vi "Day 4-2.vi"() -> ()   [LabVIEW 2019, in "Day 4.lvlib"]
uses:
  Day 4.lvlib
panel:
  out "Result":i32
  out "Winner Turn Number":i32
  out "Winner Board Status":bool[][](array[boolean])
  out "Winner Board":i32[][](array[numeric])
  in  "String":string="62,55,98,93,48,28,82,78,19,96,31,42,76,25,34,4,18,80,66,6,14,17,57,54,90,27,40,47,9,36,97,56,87,61,91,1,64,71,99,38,70,5,94,85,49,59,69,26,21,60,0,79,2,95,11,84,20,24,8,51,46,44,88,22,16,53,7,32,89,67,15,86,41,92,10,77,68,63,43,75,33,30,81,37,83,3,39,65,12,45,23,73,72,29,52,58,35,50,13,74\n\n10 83 98 12 33\n38 68  2 99 85\n16 89 54 50 97\n31  8 17 11 76\n 0 55 66 32 87\n\n77 60 61 59 16\n17 46 97  9 73\n42 82 25 32 29\n48 94 52 55 50\n95 14 67 79 34\n\n 6 31  5 74 67\n76 89 15 78 47\n54 49 62 32 38\n35 43 61 22 58\n75 97 33  8 16\n\n37 58 22 47 30\n 4 86 77 42 54\n73 94 87 34 55\n72 53 14 64 88\n23 21 36 52 66\n\n59 16 18 85 93\n96 56 50 53 94\n68 95 77  0 27\n47 30 88 46 65\n75 82 41 31 23\n\n88 96 94 75  3\n31 26 74 90 36\n59 22 41 84 54\n 6 68 37 20 93\n10 66 46  9 79\n\n33 78 12 62 73\n18 37  7 44 66\n69 15 54 53 82\n98 20 30 58 81\n56 95 36 91 99\n\n47 89 86 58 43\n49 72 84 94 51\n69 73 15 50  0\n46 81 76 31 61\n96 91 56  2 34\n\n22 91 70 68 99\n25 28  3 42  1\n21 19 79 54  4\n97 88 49  8 78\n44 98 84 83  6\n\n21  0 62  2  9\n49 81 50 66 10\n24 72 45 96  6\n51 82 17 58 91\n18 56 39 11 25\n\n22 25 42 98 93\n 1 26  0 67 65\n31 11 37  7 96\n28 17 40 79 12\n95  5  2 66 10\n\n63  8 97 64 82\n43 12 83  1 11\n69 84 74  7 59\n25 48 38 89 62\n22 93 39 71 76\n\n92 94 20 49 21\n34 41 61 98 28\n93 62 74 12 31\n63 77 87 36 55\n23  7  4 69 53\n\n61 27 76 56 12\n60  7 36 33 97\n 4 16 89 44 40\n51 43 75 79 28\n14 69 35 90  8\n\n12 34 94 77 87\n24 61 19 23 41\n75 46  9 21 64\n88 15 40 89 86\n32 47 93  3 58\n\n74 16 44 21 30\n 1 11 71 97 42\n88 59 52 28 75\n58 26 23 76  8\n33 65 80 95 14\n\n54 29  7 80 33\n20 18 82 26 93\n72  4 45 89 98\n99 16  8 22 34\n86 61 51 43 64\n\n96 20 88 78 73\n65 84 93 79 48\n25 99 13 60 41\n37 24 82  8 89\n44 10  4 58 57\n\n28 70 42 66 15\n 3 35 52 49  4\n77 23 16 30 24\n67 75  8 29 47\n39 32 80 22 55\n\n70 61  5 77  9\n 3 23 42 86 31\n99 22 41 14 17\n93 63 25 10 30\n28 52 81 89 40\n\n78 18 42 48 14\n 4 95 87 64 32\n13 10 72 90 46\n68 16 57 80 77\n50 69  5 63 96\n\n89 15 13 68 84\n37 79 56 97 34\n60 48 91 87 96\n32 25 78 55 11\n 1 67 57 93 92\n\n89 94 12 46 21\n61 67 26 40 76\n86 78  6 41 56\n35 64 28 73 98\n30 17 88 70 71\n\n37 57 36  6 32\n89 26 27 22 29\n80 49 88  0 46\n70 18 50 14 19\n34 84 79 90 98\n\n41 23 10  4 88\n26 55 17 71 15\n68 49  0 14 97\n27 61 31 74 99\n89 33 64 32  5\n\n63 44 98 56 47\n72  2 28 89 77\n36 24 26 14 21\n 7 58 32 31 86\n33  0 57 54  4\n\n 2 89 46 59  6\n62 67 84 95 98\n 8 12 75 70 88\n45 93 38 61 47\n37 55 76 82 92\n\n 2 50 19 35 34\n94  0 48 75 16\n18 92 46 38 32\n65 78 22 85 77\n69 73 88 30 60\n\n98 21 79 41 39\n64  1 91  7 44\n45 32 72 22 38\n78 28 97 69 33\n55 12 53  9 61\n\n94 39 67 82 18\n11 86 43 92  0\n44  8 66  3 91\n62 56 38 32 89\n27  2 76 90 31\n\n21 79 89 70 85\n73 76 92 15 33\n36 63 44 99 19\n35 75 88 65  3\n48 54 97 27  2\n\n35  8 51 77 29\n 1 11 38 67 99\n 2 18 94 32 24\n54 82 21 98  7\n20  0 48 83 74\n\n77 82 68 18 58\n 9 78 85 59 55\n15 73 56 46 10\n80 38 26  8 96\n41 84 35 86 12\n\n36 89 27 38 22\n53 46  5 84 90\n23  7 63 29 17\n92 41 97  0 43\n74 33 26 98 19\n\n69 40 35 84  3\n56 49 55  2 28\n85 14 50 12 27\n65 73  6 42 23\n64 68 48 62 22\n\n57  8 21 98 66\n39 92 16 95 87\n49  1 51 68 48\n46 84 17 35 80\n20 47  3 75 34\n\n23 15 77  3 91\n33 58 69 66 14\n88 47 18 16 99\n62 89 86  7 67\n90 57 35 45 29\n\n89 12 29 39 78\n26 52 10 47 97\n68 90 65 56 33\n63  8 13 27 42\n30 66 91 16 51\n\n95 91 88 40 97\n63 54 68 26 52\n56 76 78 83 62\n13 65 90 49 94\n44 74 79 48 81\n\n24 27 11 74  0\n38 56 53 25 60\n50 51 49 10 72\n76 34 52 81  9\n80 99 82  1 67\n\n90 88 71 53 26\n70 19 57 61 89\n64 30  0  9 56\n 4 21 62 38 82\n51 40 55 81 20\n\n66 14 90 76 93\n21 57 27 55 32\n22 43 67 29 81\n49 53 39 96 79\n12 48 88 63 33\n\n15  7 99 55 84\n53 80 47 75 36\n 1 22 39 91 82\n13 76 40 27 81\n57 93  8 48 28\n\n82 58  5 84 25\n61 19 83 22 44\n85  3 14 10 97\n35 26 79 20 73\n99 21 51 47 81\n\n14 32 63 18 70\n50 91 67  1 19\n 7 31 54 11  8\n51 78 35 72 77\n47 73 22  5 76\n\n 2 22 11 31 13\n66 21 83 94 87\n69  5 59 14 53\n95 41 90 43 92\n42 77 10 88  8\n\n19 88 91 43 17\n62 83 68 94 28\n73 36 58 21 66\n55 24 90 12 77\n45  6 49 27 63\n\n 6 73 93 67 18\n29 33 94 24 34\n57 96 27 37 60\n92 88 81 12 16\n49 98 30 10 72\n\n17 40 36 96 68\n91 38 88  9  6\n16 35 63 25 37\n81 43 78 64 52\n46 44 69 67 13\n\n73 36 70  5 57\n66 55 27 54 44\n20  4 68 58 26\n96 37 76 80 47\n61  2 92 71 64\n\n12 51 54 34 68\n69 99 64 44 98\n79 67 90 46 65\n31 56 45 43 30\n29 18 94 19 59\n\n70 26 91 97  0\n46 56 93 80 52\n47 25 12 31 77\n95 72 36 74  2\n38 48 68 54 73\n\n79 89 77 24 21\n30 14 46 11 38\n 3 70 84 67 48\n45 20 40 63 35\n86 74  2 76 43\n\n97 20  2 82 84\n 8 92 71 88 33\n64 26 99 93 66\n30 40 28 38 73\n62 43  5 81 22\n\n 9 47 50  8 62\n42  1 80 21 84\n66 19 32  2 30\n76 97 85 65 45\n70 26 73 72 93\n\n80 99 91 96 25\n22 76 81 62 51\n10 64 53 54 70\n55  8 49 60  1\n40 67 14 89 16\n\n92 19 72 71 40\n29 22 86 43 12\n 0 65 78 93 10\n54 55 42 61 82\n52 47 81 99 83\n\n81 22 90 66 82\n92 56 63 79 32\n72 60 30 42 20\n91 38 10 70 13\n46 52 47 11 69\n\n11 86 32 54 47\n87 38 74 41 69\n17 23 36 61 29\n97 68 62 65 83\n30  0 28 72 19\n\n55 65 28  7  5\n90 93 99 48 80\n34 94 82 19 86\n49 39 69 75 71\n 8 24 43 33 21\n\n39 70  7 56 20\n24 67 86 45  1\n33 44 83 76  2\n46 78 17 94 48\n28  4 30 77 79\n\n18 99 73 55 30\n88 92 13 97  1\n91 49 11 48 83\n94 41  5 29 72\n61 17 84 64 90\n\n 9 13 65  1 85\n11 20 30 86 84\n35 83 99 32 38\n41  7  6 49 58\n90 87 76 23 28\n\n89 16 91 76 78\n29 26 27  3 90\n42 94 43  9 57\n59 66 80 11 24\n31 53 75 28 20\n\n82 65 50 30 79\n19 53 94 17 59\n33 47 78 75  7\n84 25 80 83 76\n81 95 72 11 21\n\n28 26 52  5  3\n 4 59 51 32 41\n19 58 42 90 43\n22 89 39 40 24\n36 57 64 20  9\n\n44 65 41 79 75\n63 76  6 51 30\n12 21 73 29 97\n42 55 54 53 25\n 0 89 47 14 92\n\n56  4 60 63 21\n20 50 24 77 22\n67 66 64 91 28\n36 57 68 87 98\n 7 86 42 33 39\n\n34 15 64 46 50\n56  7 99 69 89\n83 23 57 13 70\n86 71 85 36 98\n33 76  8 54 42\n\n22 88 25 32 45\n 2 21 40 11 16\n84 37 90 27 69\n51  1 89 49 15\n72 96  0 65  6\n\n97 79 90 95  5\n14 96 57 40 30\n70 60 52 33 36\n10 86 28 51  7\n88 20 99 27 63\n\n84  6 57 66 62\n56 80 97 55 58\n92 46 81 21 26\n99 29 27 63 87\n39 20  7 35 48\n\n84 40 26  1 46\n28 42 29  5 45\n63 82 17 31  6\n30 78  2 89 67\n14 47 60 33 32\n\n40 89 32 50 90\n 1  5 83 41 77\n19 48  6 11 70\n78 56 93 36 73\n80  9 21 26 22\n\n 8 97 13  2 38\n70 61 67 55 16\n35 42 33  9 28\n26 93 86  4 65\n79 57 19 98 62\n\n42 91 75 97 66\n50 12 53 52 20\n56 70 96  5 21\n89 57 83 18 17\n77 72 95 38 98\n\n40 98 10 67 90\n16  7 75 23 13\n78 38 53 45 20\n 0 28 87 94 25\n26 83 34 56  8\n\n83 43 49 31 73\n62 54 89 12 34\n92 35 57 91 52\n58 80 20 15 90\n51 13 61  8 17\n\n19 65 73 81  5\n57 71 52 51 22\n48 53 15 34 66\n63 45 96 47 49\n58 42 56 62 76\n\n44  9 76 49 75\n78 51 87 39 54\n29 62 47 42 97\n48 73 50 89 84\n 0 40 38 20 81\n\n65 34 92 70 36\n24 54 41 31 13\n28 40 93 57 20\n19 59 89 51 77\n80 69 85 76 14\n\n67 78 60 98 88\n64 46  4 84 25\n50 87 74 56 42\n59  0  7 31 61\n93 12  9 33 32\n\n29 25 94 40 53\n49 77 65 27 18\n 5 92 75 90 47\n46 16 82  1 21\n22  3 78 13 85\n\n16  2 12 64 57\n51 28 29 46 66\n45 84 37 35 50\n90 75 34 47 39\n10 68  4 31  5\n\n30 23 47 48  7\n73 16 71 12 25\n91 53 43 79  0\n81 64 35 93 37\n83 52 87 46 85\n\n15 53 29  5 96\n23 61 52 36 83\n54 64 99 16 68\n60 82 90 58 13\n42 14 59 80 27\n\n11 54  7 24 96\n43 32  5 95 93\n22 49 85 64 40\n51 18 39 47 34\n63 21 80 75 82\n\n32  6 43 27 25\n 4 20 40 59 58\n46 47  8 65 33\n12 21 29 84  2\n86 30 26 62 37\n\n34 58 13 38 41\n40 53 52 54 94\n37 74 16 25 99\n22 62 11 61 51\n27 96  6 44  0\n\n68 87 53 96 90\n17 49 45 13 93\n21 38 62 35 27\n56  1 65 10 33\n16 48 22 47 67\n\n90 79 22 24 72\n63 65 18 12 11\n69 37  1 10 21\n73 45 64  4  8\n75 77 25 80 76\n\n84  6 82  5 21\n79 62 42 78 35\n39 41 59 65 29\n25 54  7 31 93\n43 86 15 61 96\n\n 1 80 34 86  3\n12 49 29  7 82\n16 70 23 45  2\n17 75 52 28 13\n38 25 74 77 39\n\n16 11 70 63 14\n25 61 13 84 34\n96 24 30 38 39\n75 72 59 97 91\n 8  4 62 19 58\n\n 5 66 76 33 29\n72 92  7 87 73\n68 94 93 60 61\n21  3 10 20 89\n35 47 34 48 59\n\n32 79 54 30 93\n19 45  4 26 50\n48 86 38  6 85\n25 61 66 55 51\n68 27 39 20  7\n\n40 57 61 28 85\n54 96 20 99 69\n83 33 91  2 93\n92 30 53 12 16\n35 73 58 65 98\n\n60  3 95 59 52\n75 89 91 96 92\n66  8 34 45 21\n 6 39  2 50 55\n19 26 86 12 94\n\n93 55 44 91  8\n81 89 23 77 97\n 2 92  6 76 39\n21  0 56 90 51\n16 10  5 32 66\n\n 4 62 54 89 43\n75 22 13 10 68\n91 71 69 56 96\n55 12 53 21 39\n19  5 51 70  3"
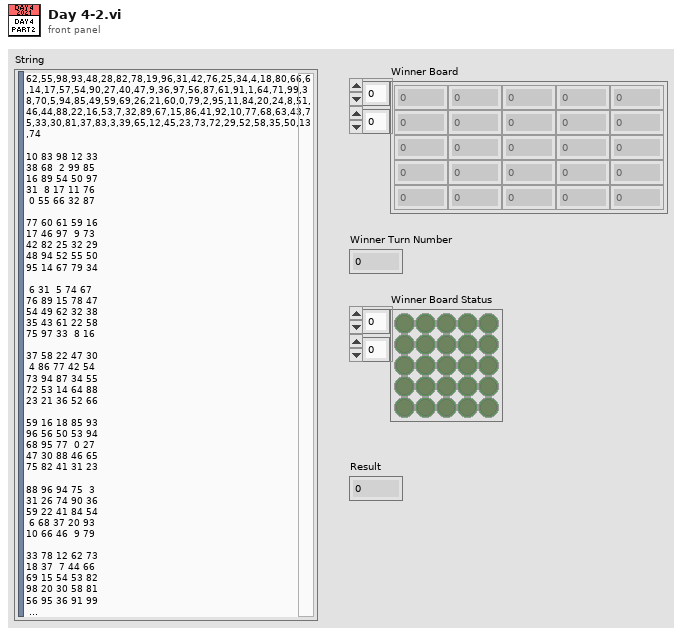
[diagram p1: front panel]
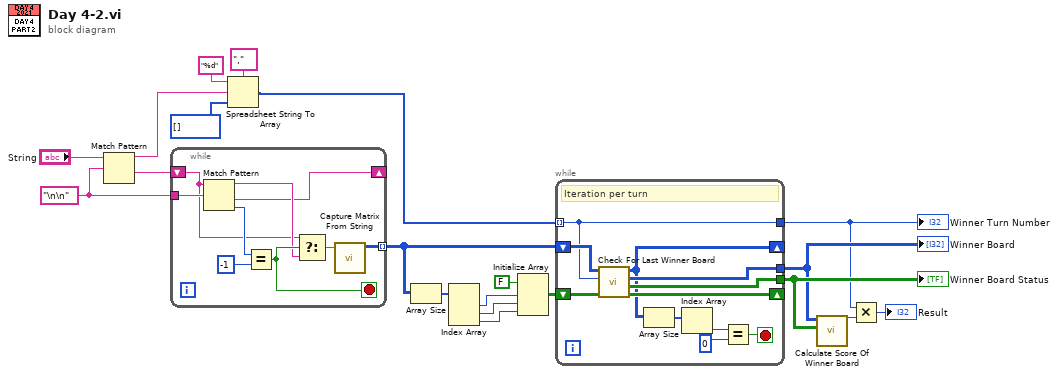
[diagram p0: block diagram]
diagram:
  w18 = "\n\n" ("regular expression")
  n1 = Match Pattern(string="String", regular expression=w18) -> (before substring=w2:string, after substring=w19:string)  [unwired: 1 in, 2 out]
  n2 = while {
    tunnel: w18 -> [w29]
    tunnel: [w26] -> w16 mode=indexing
    shift-right: [w23] -> _
    shift-left: w19 -> [w21]
    stop <- w27 stop-if-true
    n3 = Match Pattern(string=w21, regular expression=w29) -> (before substring=w24:string, after substring=w23:string, offset past match=w25:i32)  [unwired: 1 in, 1 out]
    n4 = Equal?(x=w25, y=-1) -> (x = y?=w27:bool)
    n5 = Select(t=w21, s=w27, f=w24) -> (s? t:f=w22:string)
    n6 = call "Capture Matrix From String.vi"("String"=w22) -> ("Matrix"=w26:i32[][])  [unwired: 10 in]
  }
  n7 = Spreadsheet String To Array(delimiter (Tab)=",", format string="%d", spreadsheet string=w2, array type (2D Dbl)=i32[] []) -> (array=w1:i32[])
  n8 = Array Size(array=w16) -> (size(s)=w15:i32[])
  n9 = Index Array(array=w15) -> (element #1=w14:i32, element #2=w13:i32, element #3=w12:i32)  [unwired: 3 in]
  n10 = Initialize Array(FALSE, w14, w13, w12) -> (w11:bool[][][])
  n11 = while {
    tunnel: w1 -> [w39] mode=indexing
    shift-right: [w35] -> _
    shift-left: w11 -> [w38]
    tunnel: [w37] -> w7
    tunnel: [w36] -> w10
    tunnel: [w39] -> w6
    shift-right: [w33] -> _
    shift-left: w16 -> [w40]
    stop <- w30 stop-if-true
    # "Iteration per turn"
    n12 = call "Check For Last Winner Board.vi"("Matrixes Status In"=w38, "Turn Number"=w39, "Boards"=w40) -> ("Matrixes Status Out"=w35:bool[][][], "Winner Board Status"=w36:bool[][], "Winner Board"=w37:i32[][], "Boards Without Winner"=w33:i32[][][])  [unwired: 5 in]
    n13 = Array Size(array=w33) -> (size(s)=w32:i32[])
    n14 = Index Array(array=w32) -> (element=w34:i32)  [unwired: 1 in]
    n15 = Equal?(x=w34, y=0) -> (x = y?=w30:bool)
  }
  "Winner Board" <- w7
  "Winner Board Status" <- w10
  "Winner Turn Number" <- w6
  n16 = call "Calculate Score Of Winner Board.vi"("Winner Board Status"=w10, "Winner Board"=w7) -> ("Score"=w9:i32)  [unwired: 9 in]
  n17 = Multiply(x=w6, y=w9) -> (x*y=→"Result":i32)
